vi "CTRE_Create_SensoredGearbox.vi"   [LabVIEW 2016]
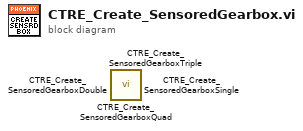
[diagram p0: block diagram]
diagram:
  n1 = call <vilib>:"CTRE_Create_SensoredGearboxQuad.vi"() -> ()  [unwired: 15 in, 1 out]
  n2 = call <vilib>:"CTRE_Create_SensoredGearboxTriple.vi"() -> ()  [unwired: 15 in, 1 out]
  n3 = call <vilib>:"CTRE_Create_SensoredGearboxDouble.vi"() -> ()  [unwired: 15 in, 1 out]
  n4 = call <vilib>:"CTRE_Create_SensoredGearboxSingle.vi"() -> ()  [unwired: 15 in, 1 out]
